vi "主界面Z020.vi"() -> ()   [LabVIEW 2013]
uses:
  <vilib>/Utility/file.llb/Read From Spreadsheet File (string).vi
  <vilib>/Utility/error.llb/whitespace.ctl
panel:
  out "判断是否合格":bool=TRUE
  out "员工ID":string
  out "涂脂工步号":dbl
  out "涂脂操作状态":string
  out "本序已做":bool
  out "B010，B020异常":bool
  out "B010有不合格项":bool
  out "B010正常状态":bool
  out "B020有不合格项":bool
  out "B020正常状态":bool
  out "上序不合格":bool
  out "上序合格":bool
  out "FGCS":string
  out "KSSJ":string
  out "RFID Z020":string
  out "读取缓冲区":string
  out "错误输出":errorcluster
  out "芯片ID":string
  out "本序不合格":bool
  out "权限":string
  out "本序合格":bool
  in  "停止":bool
  in  "自动工步号":dbl
  out "产品选型":dbl
  out "操作状态":string
  in  "联线按钮":bool
  in  "选项卡控件":enum32{"自动界面", "手动界面"}(tab)
  in  "人工判断不合格":bool
  out "拧紧NOK":bool
  out "拧紧OK":bool
  out "扭矩（NM）":string
  out "角度(度)":string
  in  "推齿条气缸进":bool
  in  "推齿条气缸退":bool
  in  "上阻挡器放行":bool
  in  "下阻挡器放行":bool
  in  "顶升气缸上升":bool
  in  "顶升气缸下降":bool
  in  "手动涂脂":bool
  out "气缸左位":bool
  out "气缸A上位":bool
  out "上工位检测":bool
  out "通讯状态":bool
  out "急停按钮":bool
  out "取轴承A监控":bool
  out "涂脂监控":bool
  out "气缸右位":bool
  out "气缸A下位":bool
  out "本工位检测":bool
  out "联线状态":bool
  out "光幕保护":bool
  out "取轴承B监控":bool
  out "气缸B上位":bool
  out "气压报警":bool
  out "下工位检测":bool
  out "取挡圈监控":bool
  out "RFID触发":bool
  out "装轴承A监控":bool
  out "气缸B下位":bool
  out "顶升下位":bool
  out "顶升上位":bool
  out "取油封监控":bool
  out "RFID完成":bool
  out "装轴承B监控":bool
  out "员工姓名":string
  in  "型号选择":u16(ring)=1 items=["J709", "J706", "J728"]
  in  "参数加载":bool
  out "产品ID":string
  # "芜湖机械转向器装配线"
  # "Z020装齿轮轴及调整螺塞总成"
  # "Q14070机械转向器装配线"
  # "湖北唯思凌科装备制造有限公司 设计开发 (C)2015"
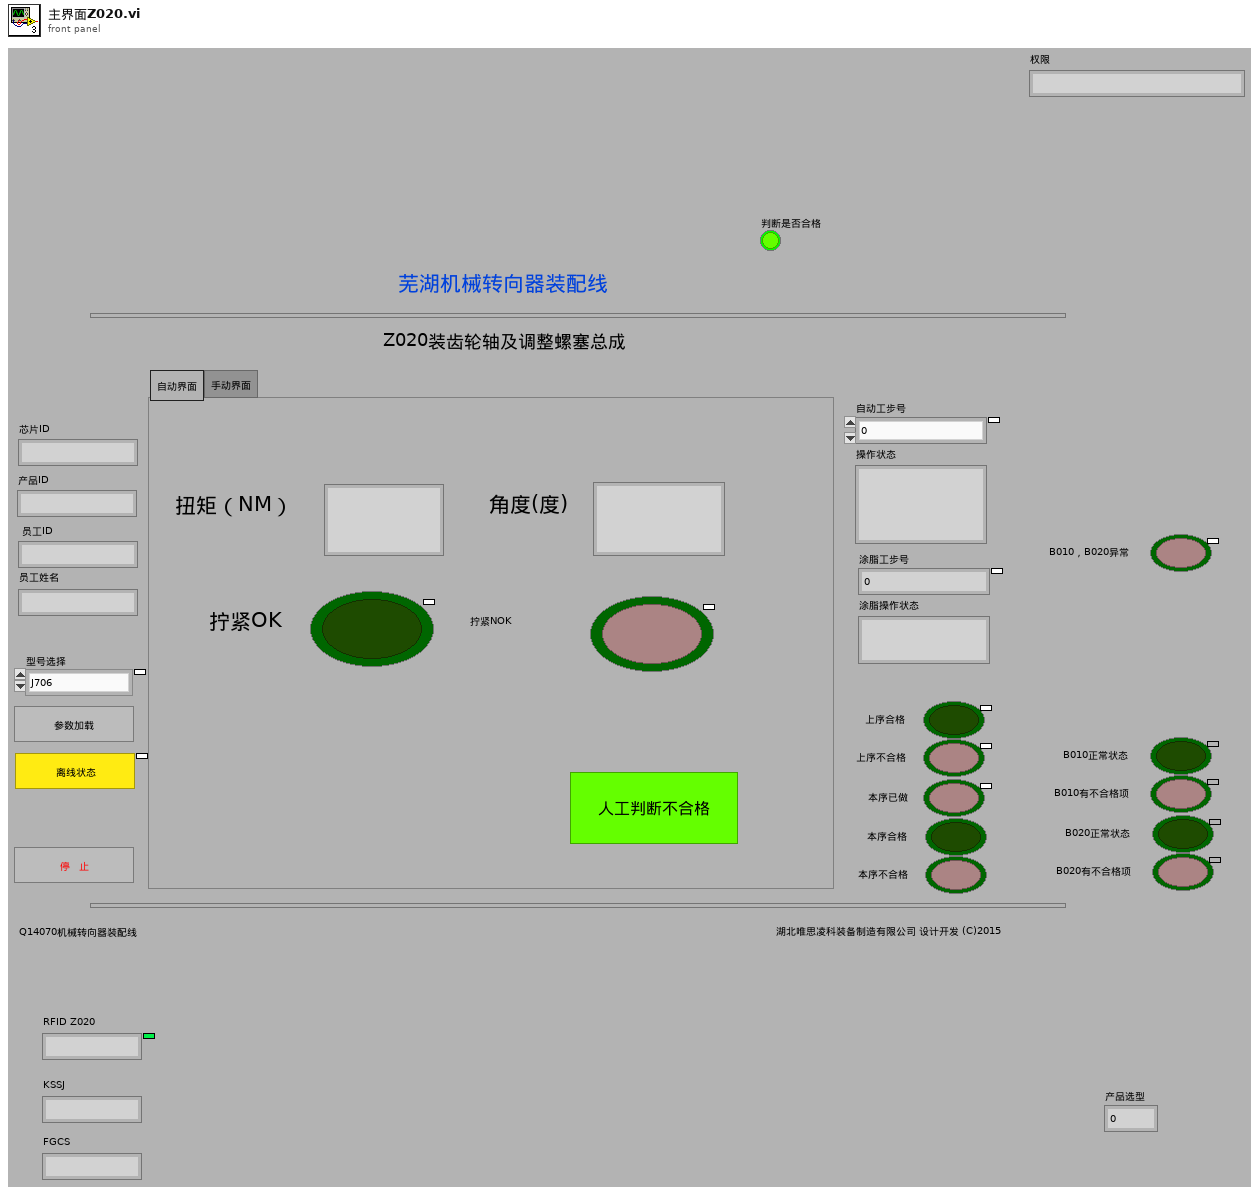
[diagram p1: front panel]
types:
  T1 = typedef "whitespace.ctl" = u16
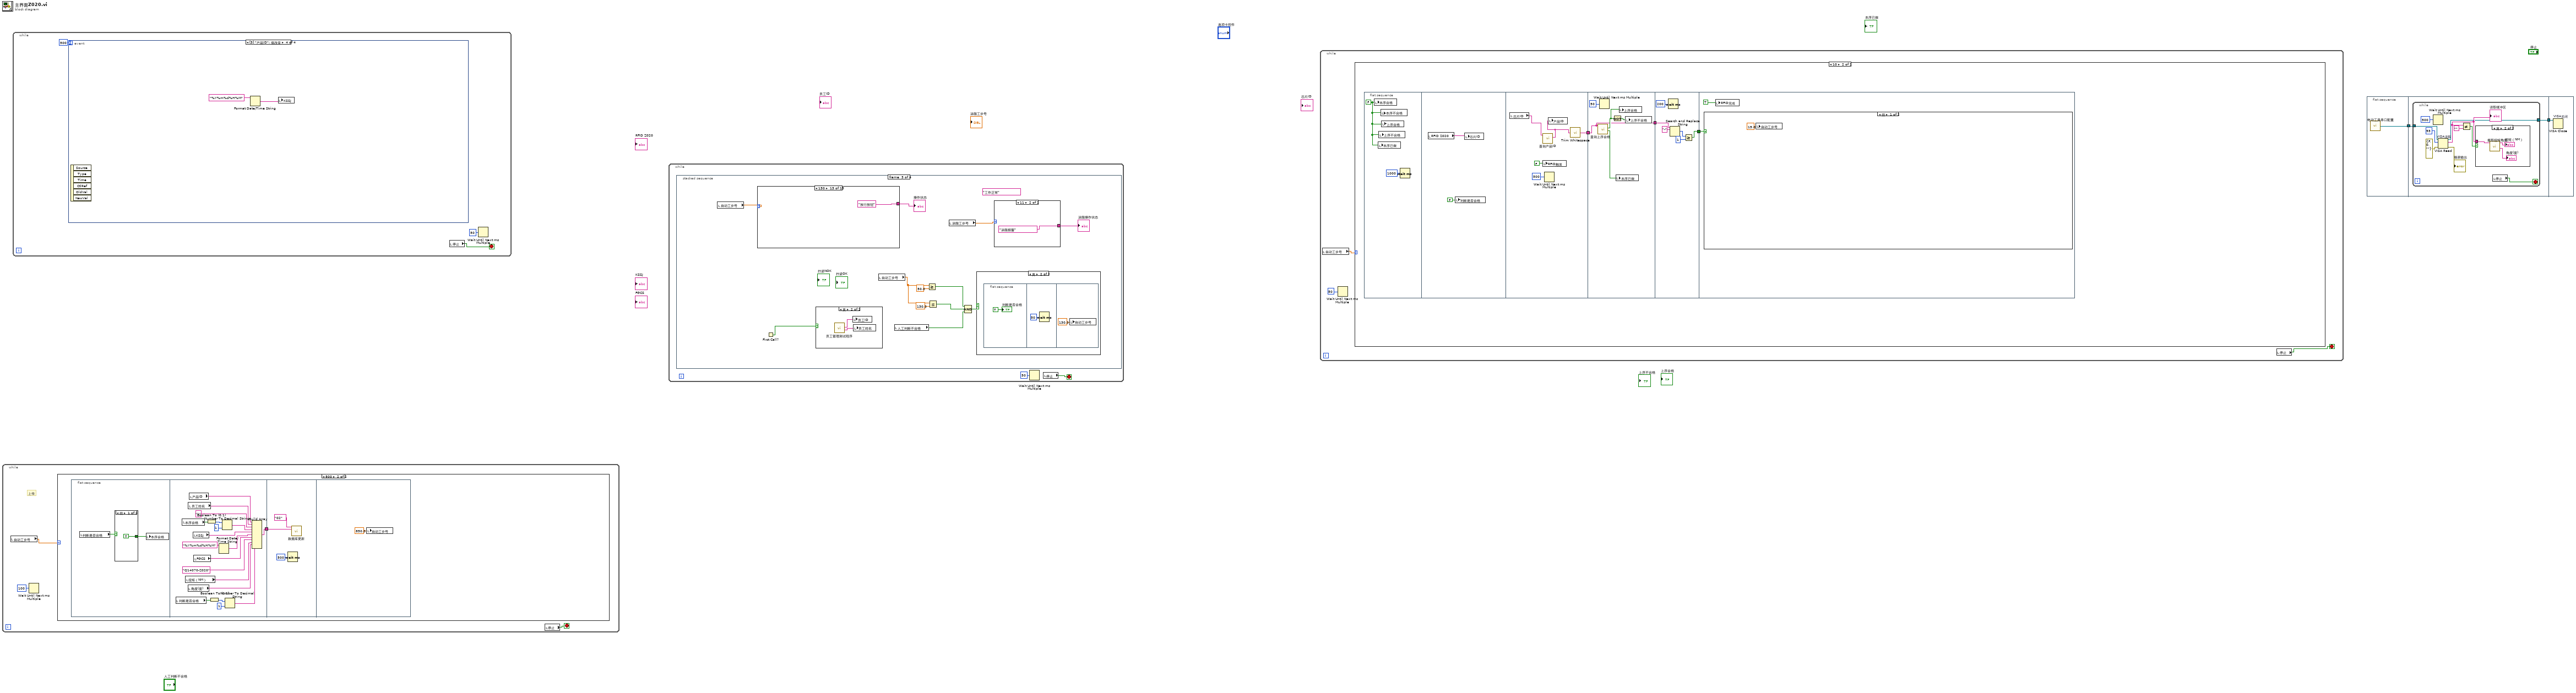
[diagram p0: block diagram]
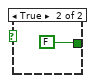
[diagram p3: hidden frame]
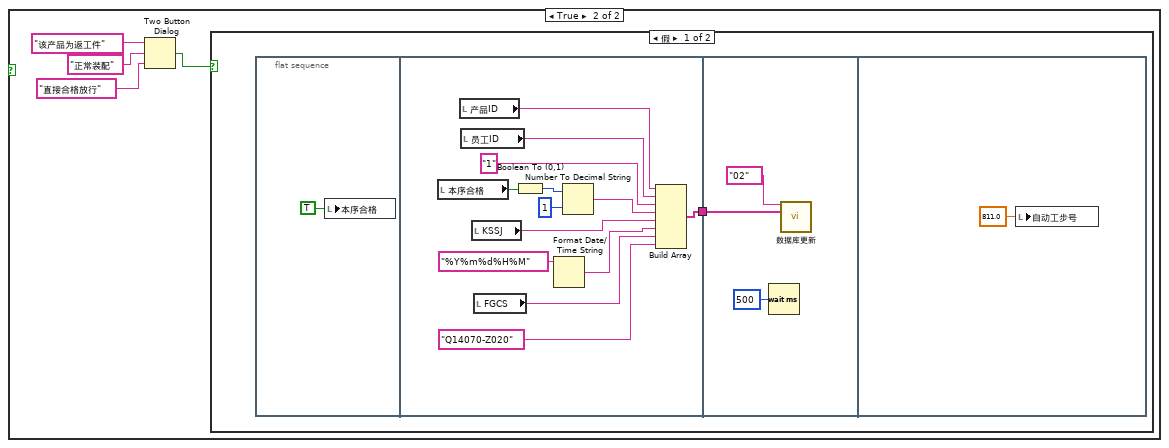
[diagram p6: hidden frame]
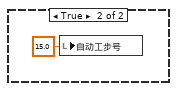
[diagram p7: hidden frame]
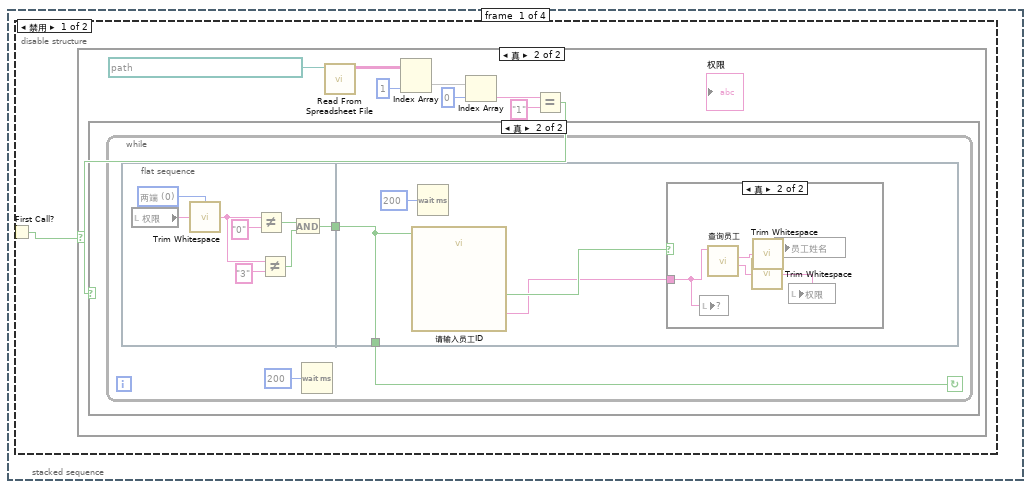
[diagram p8: hidden frame]
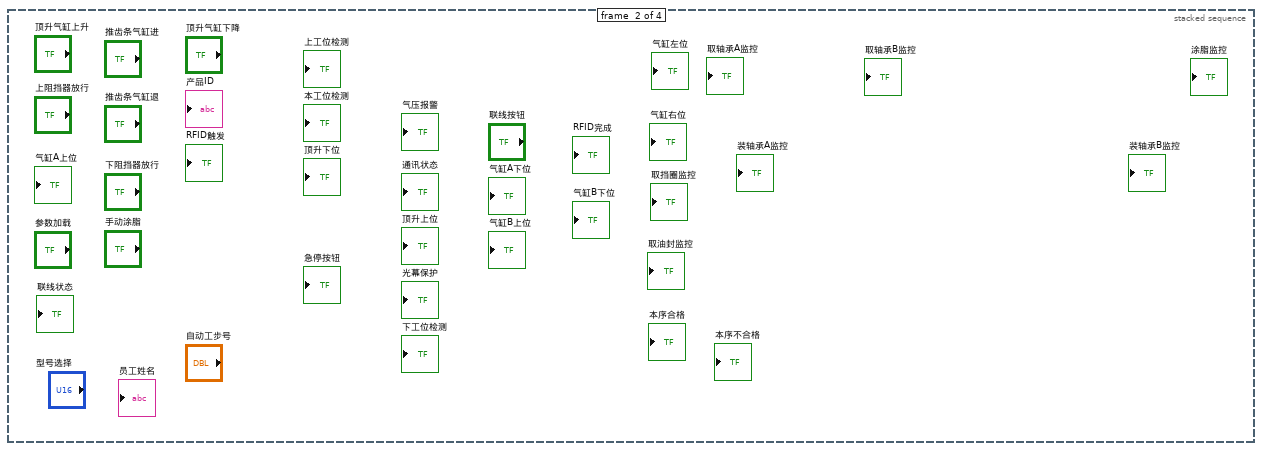
[diagram p13: hidden frame]
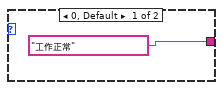
[diagram p15: hidden frame]
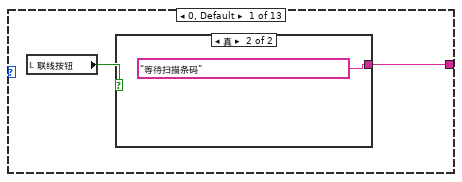
[diagram p17: hidden frame]
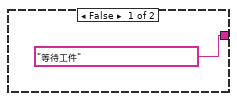
[diagram p18: hidden frame]
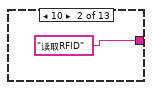
[diagram p19: hidden frame]
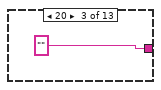
[diagram p20: hidden frame]
diagram:
  n1 = while {
    stop <- w5 stop-if-true
    # "上传"
    n2 = local read "自动工步号"() -> (w3:dbl)
    n3 = Wait Until Next ms Multiple(millisecond multiple=u32 100 ("毫秒倍数")) -> ()  [unwired: 1 out]
    n4 = case shown="800" w3 {
      frame 0, Default {
      }
      frame 800 {
        n5 = flat-sequence {
          tunnel: [w16] -> w6
          tunnel: w6 -> [w31]
          frame #0 {
            n6 = local read "判断是否合格"() -> (w8:bool)
            n7 = case shown="假" w8 {
              tunnel: [TRUE FALSE] -> w7
              frame False {
              }
              frame True {
              }
            }
            n8 = local write "本序合格"(w7) -> ()
          }
          frame #1 {
            n9 = local read "判断是否合格"() -> (w12:bool)
            n10 = local read "本序合格"() -> (w26:bool)
            n11 = local read "扭矩（NM）"() -> (w18:string)
            n12 = local read "角度(度)"() -> (w17:string)
            n13 = local read "员工姓名"() -> (w25:string)
            n14 = local read "产品ID"() -> (w15:string)
            n15 = local read "KSSJ"() -> (w22:string)
            n16 = local read "FGCS"() -> (w20:string)
            n17 = Boolean To (0,1)(Boolean=w26) -> (0, 1=w28:i16)
            n18 = Boolean To (0,1)(Boolean=w12) -> (0, 1=w13:i16)
            n19 = Format Date/Time String(time format string (%c)="%Y%m%d%H%M" ("时间格式字符串(%c)")) -> (date/time string=w21:string)  [unwired: 2 in]
            n20 = Number To Decimal String(number=w28, width (-)=i16 1 ("宽度(-)")) -> (decimal integer string=w23:string)
            n21 = Number To Decimal String(number=w13, width (-)=i16 1 ("宽度(-)")) -> (decimal integer string=w11:string)
            n22 = Build Array(w15, w25, "1", w23, w22, w21, w20, "Q14070-Z020", w18, w17, w11) -> (w16:string[])
          }
          frame #2 {
            n23 = Wait (ms)(milliseconds to wait=u32 500 ("等待时间（毫秒）")) -> ()  [unwired: 1 out]
            n24 = call "数据库更新.vi"("设备号"="02", "数据"=w31) -> ()  [unwired: 13 in, 1 out]
          }
          frame #3 {
            n25 = local write "自动工步号"(850.0 ("自动工步号")) -> ()
          }
        }
      }
    }
    n26 = local read "停止"() -> (w5:bool)
  }
  n27 = while {
    stop <- w34 stop-if-true
    n28 = event shown="[3] \"产品ID\": 值改变" {
      selector: _ -> [_ _ _ _]
      dyn-events: _ -> [_ _ _ _]
      timeout: 500 -> [_ _ _ _]
      event Timeout {
        n29 = event-data() -> ()  [unwired: 3 out]
      }
      event "参数加载": Value Change {
        n30 = event-data() -> ()  [unwired: 7 out]
      }
      event "停止": Value Change {
        n31 = event-data() -> ()  [unwired: 7 out]
        n32 = flat-sequence {
          frame #0 {
          }
          frame #1 {
            n33 = Wait Until Next ms Multiple(millisecond multiple=u32 1000 ("毫秒倍数")) -> ()  [unwired: 1 out]
          }
          frame #2 {
            n34 = Quit LabVIEW(quit? (T)=TRUE ("停止？(T)")) -> ()
          }
        }
      }
      event "产品ID": Value Change {
        n35 = event-data() -> ()  [unwired: 7 out]
        n36 = Format Date/Time String ("格式化日期/时间字符串")(time format string (%c)="%Y%m%d%H%M" ("时间格式字符串(%c)")) -> (date/time string=w39:string)  [unwired: 2 in]
        n37 = local write "KSSJ"(w39) -> ()
      }
    }
    n38 = local read "停止"() -> (w34:bool)
    n39 = Wait Until Next ms Multiple(millisecond multiple=u32 50 ("毫秒倍数")) -> ()  [unwired: 1 out]
  }
  n40 = while {
    stop <- w41 stop-if-true
    n41 = stacked-sequence {
      frame #0 {
        n42 = disable-structure shown="禁用" {
          frame Disabled {
            n43 = First Call?() -> (First Call?: T/F=w43:bool)
            n44 = case shown="真" w43 {
              frame False {
              }
              frame True {
                n45 = call-poly <vilib>:"Read From Spreadsheet File.vi"("file path (dialog if empty)"=path "\\\\Q113600\\参数/00/管理策略.txt" ("基路径")) -> ("all rows"=w46:string[][])  [unwired: 3 in, 7 out]
                n46 = Index Array(array=w46, index (col)=1 ("索引 (行)")) -> (element=w47:string[])  [unwired: 1 in]
                n47 = Index Array(array=w47, index=0 ("索引")) -> (element=w49:string)
                n48 = Equal?(x=w49, y="1") -> (x = y?=w51:bool)
                n49 = case shown="真" w51 {
                  frame False {
                  }
                  frame True {
                    n50 = while {
                      stop <- w53 continue-if-true
                      n51 = flat-sequence {
                        tunnel: [w59] -> w54
                        tunnel: w54 -> [w63]
                        tunnel: [w63] -> w53
                        frame #0 {
                          w57 = T1 0 items=["两端", "字符串首端", "字符串末端"] ("location (both)")
                          n52 = local read "权限"() -> (w55:string)
                          n53 = call <vilib>:"Trim Whitespace.vi"("string"=w55, "location (both)"=w57) -> ("trimmed string"=w56:string)
                          n54 = Not Equal?(x=w56, y="0") -> (x != y?=w58:bool)
                          n55 = Not Equal?(x=w56, y="3") -> (x != y?=w62:bool)
                          n56 = And(x=w58, y=w62) -> (x .and. y?=w59:bool)
                        }
                        frame #1 {
                          n57 = call "请输入员工ID"("Enable"=w63) -> ("请输入员工ID"=w64:string, "确定"=w65:bool)  [unwired: 1 in, 16 out]
                          n58 = Wait (ms)(milliseconds to wait=u32 200 ("等待时间（毫秒）")) -> ()  [unwired: 1 out]
                          n59 = case shown="真" w65 {
                            tunnel: w64 -> [_ w67]
                            frame False {
                            }
                            frame True {
                              n60 = local write item#-1(w67) -> ()
                              n61 = call "查询员工.vi"("员工ID"=w67) -> ("权限"=w70:string, "姓名"=w71:string)  [unwired: 7 in, 2 out]
                              n62 = call <vilib>:"Trim Whitespace.vi"("string"=w70) -> ("trimmed string"=w69:string)  [unwired: 1 in]
                              n63 = call <vilib>:"Trim Whitespace.vi"("string"=w71) -> ("trimmed string"=w68:string)  [unwired: 1 in]
                              n64 = local write "员工姓名"(w68) -> ()
                              n65 = local write "权限"(w69) -> ()
                            }
                          }
                        }
                      }
                      n66 = Wait (ms)(milliseconds to wait=u32 200 ("等待时间（毫秒）")) -> ()  [unwired: 1 out]
                    }
                  }
                }
              }
            }
          }
          frame Enabled {
          }
        }
      }
      frame #1 {
      }
      frame #2 {
        (unwired) "工作正常"
        n67 = local read "自动工步号"() -> (w83:dbl)
        n68 = case shown="130" w83 {
          tunnel: [w92 "读取RFID" ("工步操作状态") "" ("工步操作状态") "" ("工步操作状态") "涂脂按钮涂脂" ("工步操作状态") "确认保护套在位，记号笔在位，按启动按钮" ("工步操作状态") "输入轴检测" ("工步操作状态") "取保护套" ("工步操作状态") "拧紧螺塞" ("工步操作状态") "放回保护套" ("工步操作状态") "取记号笔" ("工步操作状态") "放回记号笔" ("工步操作状态") "放行按钮" ("工步操作状态")] -> w82
          frame 0, Default {
            n69 = local read "联线按钮"() -> (w91:bool)
            n70 = case shown="真" w91 {
              tunnel: ["等待工件" ("工步操作状态") "等待扫描条码" ("工步操作状态")] -> w92
              frame False {
              }
              frame True {
              }
            }
          }
          frame 10 {
          }
          frame 20 {
          }
          frame 30 {
          }
          frame 50 {
          }
          frame 70 {
          }
          frame 85 {
          }
          frame 90 {
          }
          frame 100 {
          }
          frame 110 {
          }
          frame 115 {
          }
          frame 116 {
          }
          frame 130 {
          }
        }
        "操作状态" <- w82
        n71 = First Call?() -> (First Call?: T/F=w81:bool)
        n72 = case shown="真" w81 {
          frame False {
          }
          frame True {
            n73 = call "员工管理测试程序.vi"() -> ("员工姓名"=w90:string, "员工ID"=w89:string)  [unwired: 10 in]
            n74 = local write "员工ID"(w89) -> ()
            n75 = local write "员工姓名"(w90) -> ()
          }
        }
        n76 = local read "自动工步号"() -> (w77:dbl)
        n77 = local read "人工判断不合格"() -> (w75:bool)
        n78 = Greater Or Equal?(x=w77, y=50.0) -> (x >= y?=w72:bool)
        n79 = Less Or Equal?(x=w77, y=130.0) -> (x <= y?=w73:bool)
        n80 = local read "涂脂工步号"() -> (w80:dbl)
        n81 = Compound Arithmetic op=AND(w72, w73, w75) -> (w74:bool)
        n82 = case shown="真" w74 {
          frame False {
          }
          frame True {
            n83 = flat-sequence {
              frame #0 {
                "判断是否合格" <- TRUE ("本序合格")
              }
              frame #1 {
                n84 = Wait (ms)(milliseconds to wait=u32 50 ("等待时间（毫秒）")) -> ()  [unwired: 1 out]
              }
              frame #2 {
                n85 = local write "自动工步号"(130.0 ("自动工步号")) -> ()
              }
            }
          }
        }
        n86 = case shown="11" w80 {
          tunnel: ["工作正常" "涂脂报警"] -> w79
          frame 0, Default {
          }
          frame 11 {
          }
        }
        "涂脂操作状态" <- w79
      }
      frame #3 {
        n87 = flat-sequence {
          tunnel: [w113] -> w109
          tunnel: [w112] -> w107
          tunnel: w109 -> [w118]
          tunnel: [w117] -> w108
          tunnel: w107 -> [w117]
          tunnel: w108 -> [w119]
          frame #0 {
            n88 = First Call?() -> (First Call?: T/F=w110:bool)
            n89 = case shown="真" w110 {
              frame False {
              }
              frame True {
                n90 = local write "B010，B020异常"(FALSE ("B010，B020异常")) -> ()
              }
            }
          }
          frame #1 {
            n91 = local read "B010有不合格项"() -> (w113:bool)
            n92 = local read "B020有不合格项"() -> (w112:bool)
            n93 = Or ("或")(x=w113, y=w112) -> (x .or. y?=w114:bool)
            n94 = case shown="真" w114 {
              frame False {
                n95 = local write "B010，B020异常"(FALSE ("B010，B020异常")) -> ()
              }
              frame True {
                n96 = local write "B010，B020异常"(TRUE ("B010，B020异常")) -> ()
              }
            }
          }
          frame #2 {
            n97 = case shown="真" w118 {
              frame False {
              }
              frame True {
                n98 = call "显示对话框信息"() -> ()  [unwired: 10 in, 2 out]
              }
            }
          }
          frame #3 {
            n99 = case shown="真" w119 {
              frame False {
              }
              frame True {
                n100 = call "显示对话框信息2"() -> ()  [unwired: 10 in, 2 out]
              }
            }
          }
        }
      }
    }
    n101 = Wait Until Next ms Multiple(millisecond multiple=u32 50 ("毫秒倍数")) -> ()  [unwired: 1 out]
    n102 = local read "停止"() -> (w41:bool)
  }
  n103 = while {
    stop <- w121 stop-if-true
    n104 = local read "自动工步号"() -> (w120:dbl)
    n105 = Wait Until Next ms Multiple(millisecond multiple=u32 50 ("毫秒倍数")) -> ()  [unwired: 1 out]
    n106 = case shown="10" w120 {
      frame 0, Default {
      }
      frame 10 {
        n107 = flat-sequence {
          tunnel: [w132] -> w125
          tunnel: w125 -> [w136]
          tunnel: [w136] -> w124
          tunnel: w124 -> [w144]
          tunnel: [w140] -> w123
          tunnel: w123 -> [w146]
          frame #0 {
            w127 = FALSE ("本序合格")
            n108 = local write "本序合格"(w127) -> ()
            n109 = local write "本序已做"(w127) -> ()
            n110 = local write "上序不合格"(w127) -> ()
            n111 = local write "本序不合格"(w127) -> ()
            n112 = local write "上序合格"(w127) -> ()
            n113 = Wait (ms)(milliseconds to wait=u32 1000 ("等待时间（毫秒）")) -> ()  [unwired: 1 out]
          }
          frame #1 {
            n114 = local read "RFID Z020"() -> (w129:string)
            n115 = local write "判断是否合格"(FALSE ("判断是否合格")) -> ()
            n116 = local write "芯片ID"(w129) -> ()
          }
          frame #2 {
            n117 = local read "芯片ID"() -> (w130:string)
            n118 = local write "RFID触发"(FALSE ("RFID读取触发")) -> ()
            n119 = call "查询产品ID.vi"("芯片编码"=w130) -> ("产品ID"=w131:string)  [unwired: 8 in, 2 out]
            n120 = Wait Until Next ms Multiple(millisecond multiple=u32 500 ("毫秒倍数")) -> ()  [unwired: 1 out]
            n121 = local write "产品ID"(w131) -> ()
            n122 = call <vilib>:"Trim Whitespace.vi"("string"=w131) -> ("trimmed string"=w132:string)  [unwired: 1 in]
          }
          frame #3 {
            n123 = call "查询上序合格.vi"("产品ID"=w136) -> ("本序已做"=w135:bool, "上序合格"=w137:bool)  [unwired: 8 in, 1 out]
            n124 = Wait Until Next ms Multiple(millisecond multiple=u32 50 ("毫秒倍数")) -> ()  [unwired: 1 out]
            n125 = Not(x=w137) -> (.not. x?=w138:bool)
            n126 = local write "本序已做"(w135) -> ()
            n127 = local write "上序合格"(w137) -> ()
            n128 = local write "上序不合格"(w138) -> ()
          }
          frame #4 {
            n129 = Wait (ms)(milliseconds to wait=u32 200 ("等待时间（毫秒）")) -> ()  [unwired: 1 out]
            n130 = Search and Replace String(input string=w144, search string="-" ("搜索字符串")) -> (number of replacements=w142:i32)  [unwired: 6 in, 3 out]
            n131 = Greater Or Equal?(x=w142, y=1) -> (x >= y?=w140:bool)
          }
          frame #5 {
            n132 = case shown="假" w146 {
              frame False {
                n133 = local write "自动工步号"(15.0 ("工步号")) -> ()
              }
              frame True {
                n134 = Two Button Dialog(message="该产品为返工件" ("消息"), 1:"直接合格放行" ("F按钮名称（“取消”）"), 2:"正常装配" ("T按钮名称（“确定”）")) -> (T button?=w149:bool)
                n135 = case shown="假" w149 {
                  frame False {
                    n136 = flat-sequence {
                      tunnel: [w156] -> w153
                      tunnel: w153 -> [w169]
                      frame #0 {
                        n137 = local write "本序合格"(TRUE ("本序合格")) -> ()
                      }
                      frame #1 {
                        n138 = local read "本序合格"() -> (w164:bool)
                        n139 = local read "产品ID"() -> (w155:string)
                        n140 = local read "员工ID"() -> (w163:string)
                        n141 = local read "KSSJ"() -> (w160:string)
                        n142 = local read "FGCS"() -> (w158:string)
                        n143 = Boolean To (0,1)(Boolean=w164) -> (0, 1=w166:i16)
                        n144 = Format Date/Time String(time format string (%c)="%Y%m%d%H%M" ("时间格式字符串(%c)")) -> (date/time string=w159:string)  [unwired: 2 in]
                        n145 = Number To Decimal String(number=w166, width (-)=i16 1 ("宽度(-)")) -> (decimal integer string=w161:string)
                        n146 = Build Array(w155, w163, "1", w161, w160, w159, w158, "Q14070-Z020") -> (w156:string[])
                      }
                      frame #2 {
                        n147 = Wait (ms)(milliseconds to wait=u32 500 ("等待时间（毫秒）")) -> ()  [unwired: 1 out]
                        n148 = call "数据库更新.vi"("设备号"="02", "数据"=w169) -> ()  [unwired: 13 in, 1 out]
                      }
                      frame #3 {
                        n149 = local write "自动工步号"(811.0 ("自动工步号")) -> ()
                      }
                    }
                  }
                  frame True {
                    n150 = local write "自动工步号"(15.0 ("工步号")) -> ()
                  }
                }
              }
            }
            n151 = local write "RFID完成"(TRUE ("RFID读取完成")) -> ()
          }
        }
      }
    }
    n152 = local read "停止"() -> (w121:bool)
  }
  n153 = flat-sequence {
    tunnel: [w173] -> w2
    tunnel: w2 -> [w175]
    tunnel: [w174] -> w1
    tunnel: w1 -> [w189]
    frame #0 {
      n154 = call "电动工具串口配置.vi"() -> ("VISA resource name out"=w173:refnum<visa-resource-name>)  [unwired: 5 in]
    }
    frame #1 {
      n155 = while {
        tunnel: w175 -> [w185]
        tunnel: [w180] -> w174
        stop <- w177 stop-if-true
        n156 = Wait Until Next ms Multiple(millisecond multiple=u32 500 ("毫秒倍数")) -> ()  [unwired: 1 out]
        n157 = VISA Read "VISA读取"(VISA resource name=w185, byte count=u32 93 ("字节总数"), error in (no error)=errorcluster {"status"=FALSE, "code"=0, "source"=""} ("错误输入（无错误）")) -> (VISA resource name out=w180:refnum<visa-resource-name>, read buffer=w181:string, error out=→"错误输出":errorcluster)  [unwired: 1 out]
        "读取缓冲区" <- w181
        n158 = Not Equal?(x=w181, y="") -> (x != y?=w182:bool)
        n159 = case shown="真" w182 {
          tunnel: w181 -> [_ w188]
          frame False {
          }
          frame True {
            n160 = call "提取扭矩角度.vi"("字符串"=w188) -> ("角度值"=→"角度(度)":string, "扭矩值"=→"扭矩（NM）":string)  [unwired: 9 in]
          }
        }
        n161 = local read "停止"() -> (w177:bool)
      }
    }
    frame #2 {
      n162 = VISA Close "VISA关闭"(VISA resource name=w189) -> ()  [unwired: 1 in, 1 out]
    }
  }
